vi "Write Netway Data.vi"(4 "ZGW?":bool, 6 "In/Out":T1=enum."Output", 8 "Cal Unit":T2, 9 "Channel":T3, 10 "Verify Table":string[][](array[string]), 11 "Cal Path":path) -> ()   [LabVIEW 2013]
uses:
  Type Defs/Channel Type Def (Netway).ctl
  Type Defs/Units Type Def (Netway).ctl
  Type Defs/Input or Output Type Def.ctl
  Type Defs/Excel Driver Operator Type Def.ctl
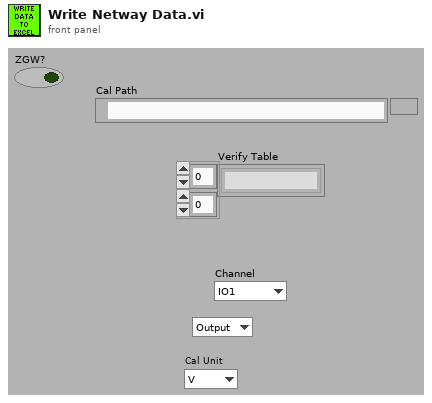
[diagram p1: front panel]
types:
  T1 = typedef "Input or Output Type Def.ctl" = enum16{"Input", "Output"}
  T2 = typedef "Units Type Def (Netway).ctl" = enum16{"V", "%", "Hz"}
  T3 = typedef "Channel Type Def (Netway).ctl" = enum16{"IO1", "IO2", "IO3", "IO4", "IO5", "IO6", "IO7", "IO8", "IO9", "IO10", "IO11", "IO12", "AIO1", "AIO2", "AIO3", "AIO4", "AIO5", "AIO6", "AIO7", "AIO8"}
  T4 = typedef "Excel Driver Operator Type Def.ctl" = enum16{"Open", "Close", "Search for String", "GetUsedRange", "Read Range", "Read Cell", "Set Range", "Set Cell"}
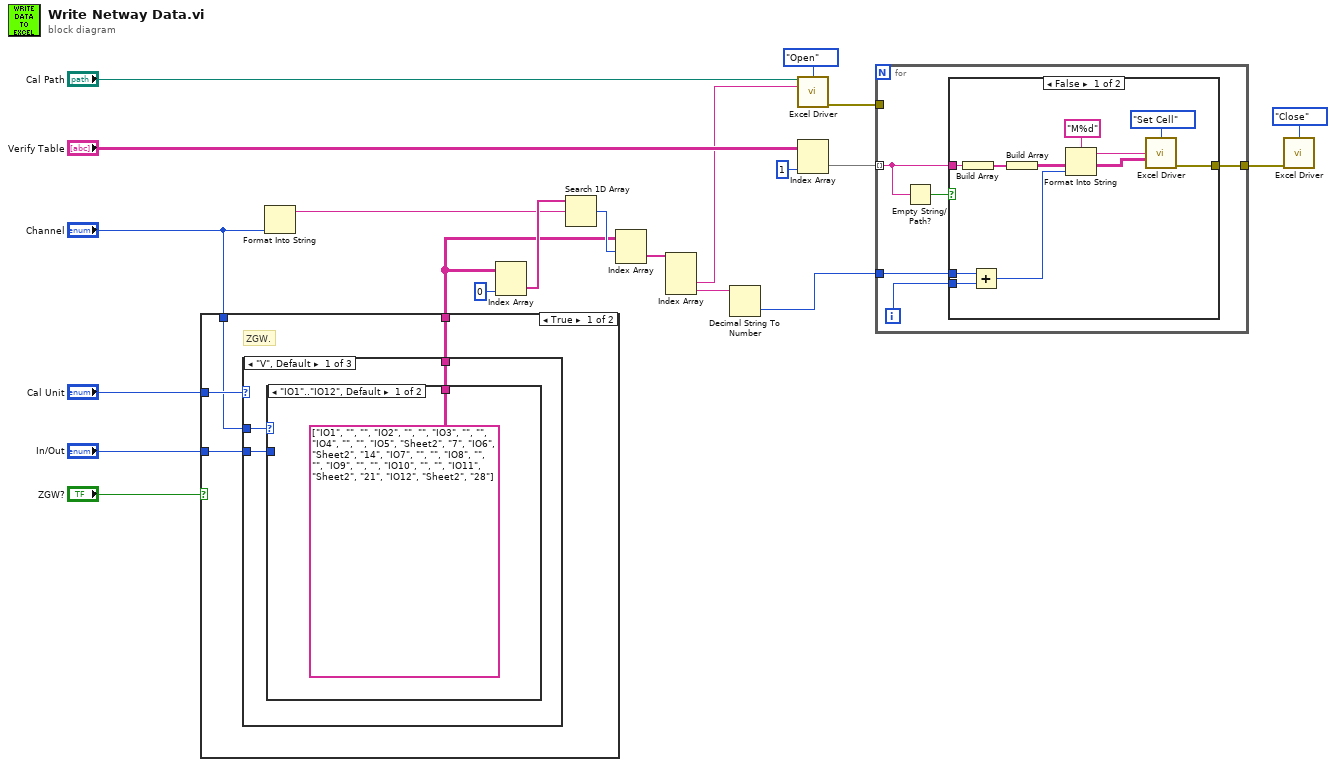
[diagram p0: block diagram]
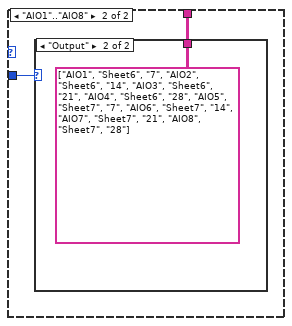
[diagram p2: hidden frame]
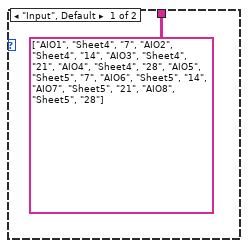
[diagram p3: hidden frame]
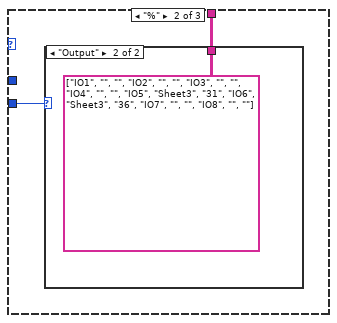
[diagram p4: hidden frame]
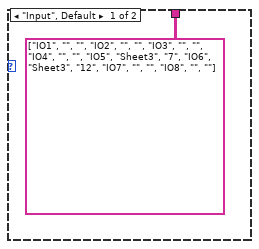
[diagram p5: hidden frame]
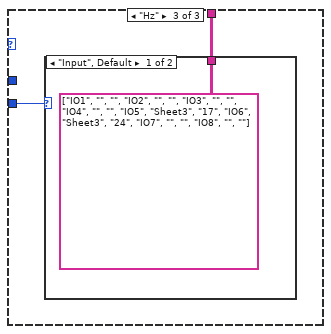
[diagram p6: hidden frame]
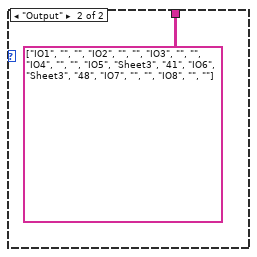
[diagram p7: hidden frame]
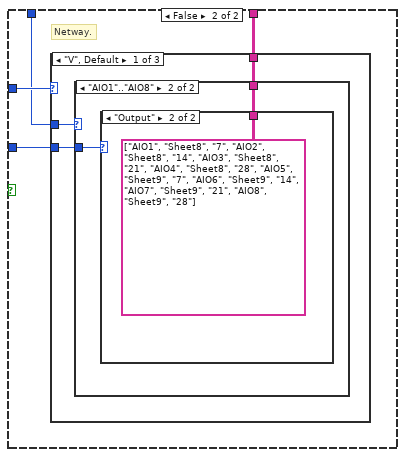
[diagram p8: hidden frame]
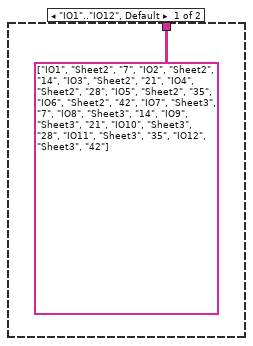
[diagram p9: hidden frame]
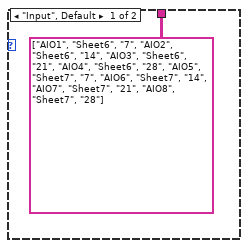
[diagram p10: hidden frame]
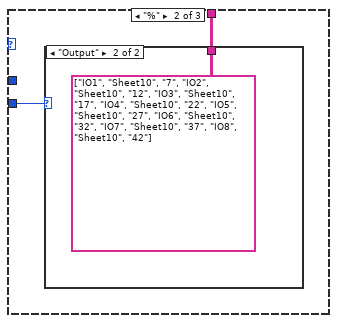
[diagram p11: hidden frame]
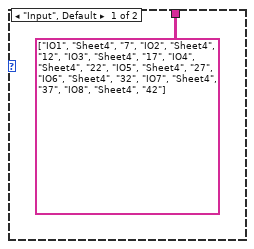
[diagram p12: hidden frame]
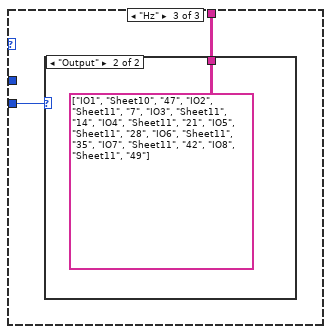
[diagram p13: hidden frame]
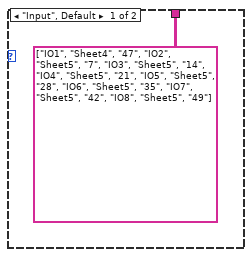
[diagram p14: hidden frame]
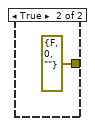
[diagram p15: hidden frame]
diagram:
  n1 = case shown="True" "ZGW?" {
    tunnel: "Cal Unit" -> [w25 w45]
    tunnel: [w24 w44] -> w5
    tunnel: "Channel" -> [w23 w43]
    tunnel: "In/Out" -> [w22 w42]
    frame True {
      # "ZGW."
      n2 = case shown="\"V\", Default" w25 {
        tunnel: [w28 w35 w39] -> w24
        tunnel: w23 -> [w27 _ _]
        tunnel: w22 -> [w26 w34 w38]
        frame "V", Default {
          n3 = case shown="\"IO1\"..\"IO12\", Default" w27 {
            tunnel: [string[][] [["IO1", "", ""], ["IO2", "", ""], ["IO3", "", ""], ["IO4", "", ""], ["IO5", "Sheet2", "7"], ["IO6", "Sheet2", "14"], ["IO7", "", ""], ["IO8", "", ""], ["IO9", "", ""], ["IO10", "", ""], ["IO11", "Sheet2", "21"], ["IO12", "Sheet2", "28"]] ("deleted portion") w31] -> w28
            tunnel: w26 -> [_ w30]
            frame "IO1".."IO12", Default {
            }
            frame "AIO1".."AIO8" {
              n4 = case shown="\"Output\"" w30 {
                tunnel: [string[][] [["AIO1", "Sheet4", "7"], ["AIO2", "Sheet4", "14"], ["AIO3", "Sheet4", "21"], ["AIO4", "Sheet4", "28"], ["AIO5", "Sheet5", "7"], ["AIO6", "Sheet5", "14"], ["AIO7", "Sheet5", "21"], ["AIO8", "Sheet5", "28"]] ("deleted portion") string[][] [["AIO1", "Sheet6", "7"], ["AIO2", "Sheet6", "14"], ["AIO3", "Sheet6", "21"], ["AIO4", "Sheet6", "28"], ["AIO5", "Sheet7", "7"], ["AIO6", "Sheet7", "14"], ["AIO7", "Sheet7", "21"], ["AIO8", "Sheet7", "28"]] ("deleted portion")] -> w31
                frame "Input", Default {
                }
                frame "Output" {
                }
              }
            }
          }
        }
        frame "%" {
          n5 = case shown="\"Output\"" w34 {
            tunnel: [string[][] [["IO1", "", ""], ["IO2", "", ""], ["IO3", "", ""], ["IO4", "", ""], ["IO5", "Sheet3", "7"], ["IO6", "Sheet3", "12"], ["IO7", "", ""], ["IO8", "", ""]] ("deleted portion") string[][] [["IO1", "", ""], ["IO2", "", ""], ["IO3", "", ""], ["IO4", "", ""], ["IO5", "Sheet3", "31"], ["IO6", "Sheet3", "36"], ["IO7", "", ""], ["IO8", "", ""]] ("deleted portion")] -> w35
            frame "Input", Default {
            }
            frame "Output" {
            }
          }
        }
        frame "Hz" {
          n6 = case shown="\"Input\", Default" w38 {
            tunnel: [string[][] [["IO1", "", ""], ["IO2", "", ""], ["IO3", "", ""], ["IO4", "", ""], ["IO5", "Sheet3", "17"], ["IO6", "Sheet3", "24"], ["IO7", "", ""], ["IO8", "", ""]] ("deleted portion") string[][] [["IO1", "", ""], ["IO2", "", ""], ["IO3", "", ""], ["IO4", "", ""], ["IO5", "Sheet3", "41"], ["IO6", "Sheet3", "48"], ["IO7", "", ""], ["IO8", "", ""]] ("deleted portion")] -> w39
            frame "Input", Default {
            }
            frame "Output" {
            }
          }
        }
      }
    }
    frame False {
      # "Netway."
      n7 = case shown="\"V\", Default" w45 {
        tunnel: [w48 w55 w59] -> w44
        tunnel: w43 -> [w47 _ _]
        tunnel: w42 -> [w46 w54 w58]
        frame "V", Default {
          n8 = case shown="\"AIO1\"..\"AIO8\"" w47 {
            tunnel: [string[][] [["IO1", "Sheet2", "7"], ["IO2", "Sheet2", "14"], ["IO3", "Sheet2", "21"], ["IO4", "Sheet2", "28"], ["IO5", "Sheet2", "35"], ["IO6", "Sheet2", "42"], ["IO7", "Sheet3", "7"], ["IO8", "Sheet3", "14"], ["IO9", "Sheet3", "21"], ["IO10", "Sheet3", "28"], ["IO11", "Sheet3", "35"], ["IO12", "Sheet3", "42"]] ("deleted portion") w51] -> w48
            tunnel: w46 -> [_ w50]
            frame "IO1".."IO12", Default {
            }
            frame "AIO1".."AIO8" {
              n9 = case shown="\"Output\"" w50 {
                tunnel: [string[][] [["AIO1", "Sheet6", "7"], ["AIO2", "Sheet6", "14"], ["AIO3", "Sheet6", "21"], ["AIO4", "Sheet6", "28"], ["AIO5", "Sheet7", "7"], ["AIO6", "Sheet7", "14"], ["AIO7", "Sheet7", "21"], ["AIO8", "Sheet7", "28"]] ("deleted portion") string[][] [["AIO1", "Sheet8", "7"], ["AIO2", "Sheet8", "14"], ["AIO3", "Sheet8", "21"], ["AIO4", "Sheet8", "28"], ["AIO5", "Sheet9", "7"], ["AIO6", "Sheet9", "14"], ["AIO7", "Sheet9", "21"], ["AIO8", "Sheet9", "28"]] ("deleted portion")] -> w51
                frame "Input", Default {
                }
                frame "Output" {
                }
              }
            }
          }
        }
        frame "%" {
          n10 = case shown="\"Output\"" w54 {
            tunnel: [string[][] [["IO1", "Sheet4", "7"], ["IO2", "Sheet4", "12"], ["IO3", "Sheet4", "17"], ["IO4", "Sheet4", "22"], ["IO5", "Sheet4", "27"], ["IO6", "Sheet4", "32"], ["IO7", "Sheet4", "37"], ["IO8", "Sheet4", "42"]] ("deleted portion") string[][] [["IO1", "Sheet10", "7"], ["IO2", "Sheet10", "12"], ["IO3", "Sheet10", "17"], ["IO4", "Sheet10", "22"], ["IO5", "Sheet10", "27"], ["IO6", "Sheet10", "32"], ["IO7", "Sheet10", "37"], ["IO8", "Sheet10", "42"]] ("deleted portion")] -> w55
            frame "Input", Default {
            }
            frame "Output" {
            }
          }
        }
        frame "Hz" {
          n11 = case shown="\"Output\"" w58 {
            tunnel: [string[][] [["IO1", "Sheet4", "47"], ["IO2", "Sheet5", "7"], ["IO3", "Sheet5", "14"], ["IO4", "Sheet5", "21"], ["IO5", "Sheet5", "28"], ["IO6", "Sheet5", "35"], ["IO7", "Sheet5", "42"], ["IO8", "Sheet5", "49"]] ("deleted portion") string[][] [["IO1", "Sheet10", "47"], ["IO2", "Sheet11", "7"], ["IO3", "Sheet11", "14"], ["IO4", "Sheet11", "21"], ["IO5", "Sheet11", "28"], ["IO6", "Sheet11", "35"], ["IO7", "Sheet11", "42"], ["IO8", "Sheet11", "49"]] ("deleted portion")] -> w59
            frame "Input", Default {
            }
            frame "Output" {
            }
          }
        }
      }
    }
  }
  n12 = Format Into String("Channel") -> (resulting string=w4:string)  [unwired: 3 in, 1 out]
  n13 = Index Array(array=w5, index (col)=0 ("disabled index (col)")) -> (element=w12:string[])  [unwired: 1 in]
  n14 = Search 1D Array(1D array=w12, element=w4) -> (index of element=w11:i32)  [unwired: 1 in]
  n15 = Index Array(array=w5, index (row)=w11) -> (element=w10:string[])  [unwired: 1 in]
  n16 = Index Array(array=w10) -> (element #2=w9:string, element #3=w8:string)  [unwired: 3 in, 1 out]
  n17 = Decimal String To Number(string=w8) -> (number=w7:i32)  [unwired: 2 in, 1 out]
  n18 = call "Excel Driver.vi"("Filename of Workbook"="Cal Path", "Operator"=Excel_Driver_Operator_Type_Def."Open", "WorkSheet Name"=w9) -> ("error out"=w17:errorcluster)  [unwired: 10 in, 2 out]
  n19 = Index Array(array="Verify Table", index (col)=1 ("disabled index (col)")) -> (element=w18:string[])  [unwired: 1 in]
  n20 = for {
    tunnel: w18 -> [w63] mode=indexing
    tunnel: w7 -> [w66]
    tunnel: w17 -> [_]
    tunnel: [w65] -> w15
    i -> [w64]
    n21 = Empty String/Path?(string/path=w63) -> (empty?=w62:bool)
    n22 = case shown="False" w62 {
      tunnel: w63 -> [w75 _]
      tunnel: w66 -> [w69 _]
      tunnel: [w68 errorcluster {"status"=FALSE, "code"=0, "source"=""} ("error out")] -> w65
      tunnel: w64 -> [w67 _]
      frame False {
        n23 = Build Array(w75) -> (w74:string[])
        n24 = Add(x=w69, y=w67) -> (x+y=w70:i32)
        n25 = Build Array(w74) -> (w73:string[][])
        n26 = Format Into String(format string="M%d", w70) -> (resulting string=w71:string)  [unwired: 2 in, 1 out]
        n27 = call "Excel Driver.vi"("Operator"=Excel_Driver_Operator_Type_Def."Set Cell", "Range String\n(Or Search String)"=w71, "Cell Values INPUT"=w73) -> ("error out"=w68:errorcluster)  [unwired: 10 in, 2 out]
      }
      frame True {
      }
    }
  }
  n28 = call "Excel Driver.vi"("Operator"=Excel_Driver_Operator_Type_Def."Close", "error in (no error)"=w15) -> ()  [unwired: 11 in, 3 out]
